vi "De Boor.vi"(6 "degree":u16, 8 "knots":dbl[](array[numeric]), 9 "spline segment idx":i32, 10 "points":dbl[][](array[numeric]), 11 "position":dbl) -> (3 "points out":dbl[][](array[numeric]))   [LabVIEW 2019]
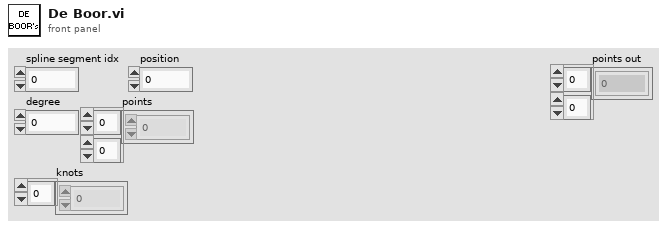
[diagram p1: front panel]
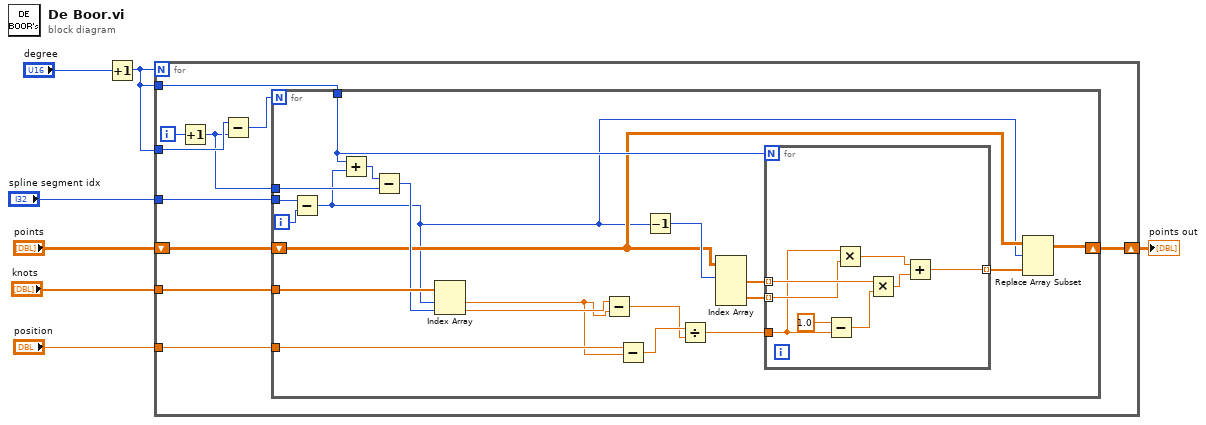
[diagram p0: block diagram]
diagram:
  n1 = Increment(x="degree") -> (x+1=w1:u16)
  n2 = for {
    N: w1 -> [_]
    tunnel: w1 -> [w9]
    tunnel: "spline segment idx" -> [w15]
    tunnel: "knots" -> [w14]
    tunnel: w1 -> [w13]
    tunnel: "position" -> [w12]
    shift-right: [w10] -> w2
    shift-left: "points" -> [w11]
    i -> [w17]
    n3 = Increment(x=w17) -> (x+1=w8:i32)
    n4 = Subtract(x=w9, y=w8) -> (x-y=w16:i32)
    n5 = for {
      N: w16 -> [_]
      tunnel: w15 -> [w37]
      tunnel: w14 -> [w36]
      tunnel: w13 -> [w26]
      tunnel: w8 -> [w34]
      tunnel: w12 -> [w31]
      shift-right: [w19] -> w10
      shift-left: w11 -> [w22]
      i -> [w20]
      n6 = Subtract(x=w37, y=w20) -> (x-y=w18:i32)
      n7 = Add(x=w26, y=w18) -> (x+y=w35:i32)
      n8 = Subtract(x=w35, y=w34) -> (x-y=w33:i32)
      n9 = Index Array(array=w36, index #1=w18, index #2=w33) -> (element #1=w30:dbl, element #2=w32:dbl)
      n10 = Subtract(x=w32, y=w30) -> (x-y=w28:dbl)
      n11 = Subtract(x=w31, y=w30) -> (x-y=w29:dbl)
      n12 = Decrement(x=w18) -> (x-1=w25:i32)
      n13 = Divide(x=w29, y=w28) -> (x/y=w27:dbl)
      n14 = Index Array(array=w22, index (row) #1=w25) -> (element #1=w24:dbl[], element #2=w23:dbl[])  [unwired: 3 in]
      n15 = for {
        N: w26 -> [_]
        tunnel: w27 -> [w41]
        tunnel: w24 -> [w44] mode=indexing
        tunnel: w23 -> [w42] mode=indexing
        tunnel: [w38] -> w21 mode=indexing
        n16 = Subtract(x=1.0, y=w41) -> (x-y=w43:dbl)
        n17 = Multiply(x=w41, y=w42) -> (x*y=w39:dbl)
        n18 = Multiply(x=w44, y=w43) -> (x*y=w40:dbl)
        n19 = Add(x=w39, y=w40) -> (x+y=w38:dbl)
      }
      n20 = Replace Array Subset(array=w22, new element=w21, index (row)=w18) -> (w19:dbl[][])  [unwired: 1 in]
    }
  }
  "points out" <- w2
